vi "Main v1.8.vi"() -> ()   [LabVIEW 2017]
doc: "v0.85:\n- Counts for rejects and total\n\nv0.5:\n\n- Added Reject to Manual Mode\n- Send reject pallet cluster during manual mode\n- Run continuous manual happens only when no error has occured"
uses:
  Controls/Main Tabs v0.1.ctl
  Controls/Auto.ctl
  RT/Controls/Auto Delays.ctl
  RT/Controls/Auto Times.ctl
  support/Controls/General Para.ctl
  Controls/UI Data.ctl
  support/Controls/Auto Stats.ctl
  Controls/Logging FGV.ctl
  support/Message Queue/Enqueue Message (Single).vi
  GV/Maintenance GV.vi
  <vilib>/Utility/error.llb/Error Cluster From Error Code.vi
  <vilib>/ErrorRing/Error Ring.xnode
  support/Message Queue/Message Queue.lvlib
  support/User Event - Stop/User Event - Stop.lvlib
panel:
  out "OEE":dbl format="%#.1f"
  out "QUA":dbl=100.0 min=0.0 max=100.0 step=0.1
  in  "Ideal Time":dbl=2.0 min=0.0 max=100.0 step=0.1
  in  "AVL":dbl=100.0 min=0.0 max=100.0 step=0.1
  out "PRF":dbl=100.0 min=0.0 max=100.0 step=0.1
  out "path":path
  in  "General Para 2":T1={"Max. Cons."=5.0, "Offset 1"=0.0, "Offset 2"=0.0, "Offset 3"=0.0, "Offset 4"=-0.6, "OutputPause"=500.0, "RejectPause"=500.0} caption="General Para" {"Offset 4" format="%.2f"; "Offset 3" format="%.2f"; "Offset 2" format="%.2f"; "Offset 1" format="%.2f"}
  in  "Auto Para 2":T2={"Agitator Delays"=[250, 600], "TF Delays"=[400, 800, 2, 8000], "Insertion Delays"=[100, 400], "Cutting Delays"=[200, 300, 50], "PF Delays"=[300, 8000], "Measur. Delays"=[200.0, 188.9, 1.0], "Reject Delays"=[500], "BF Delays"=[1000, 1000]}
  out "Shutdown?":bool
  in  "Reject Pallets":T3
  out "Date-Time":string caption="Dip-Tube Assembly Automation (HMI) v1.6"
  out "Main Tab":T4
  in  "All IOs":bool
  in  "Autocycle":T5
  in  "Manual":bool
  in  "Parameters":bool
  in  "Maintenance":bool
  in  "General Para":T1={"Max. Cons."=5.0, "Offset 1"=0.0, "Offset 2"=0.0, "Offset 3"=0.0, "Offset 4"=0.0, "OutputPause"=0.0, "RejectPause"=0.0} {"Offset 4" format="%.2f"; "Offset 3" format="%.2f"; "Offset 2" format="%.2f"; "Offset 1" format="%.2f"}
  in  "BF Para":cluster{"Delay 1":u32, "Delay 2":u32}={"Delay 1"=1000, "Delay 2"=1000}
  in  "Reject Para":cluster{"Delay":u32}={"Delay"=400}
  in  "PF Para":cluster{"Delay 1":u32, "Delay 2":u32}={"Delay 1"=1000, "Delay 2"=1000}
  in  "Tube Feeder Para":T6={"Delay"=400, "Delay 2"=250, "Max Attempts"=250, "Timeout"=8000} caption="TF Para"
  in  "Agitator Para":cluster{"Delay 1":u32, "Delay 2":u32}={"Delay 1"=400, "Delay 2"=250}
  in  "Insertion Para":cluster{"Delay 1":u32, "Delay 2":u32}={"Delay 1"=1000, "Delay 2"=1000}
  in  "Save Para":bool
  in  "Home Para":bool
  in  "Cutting Para":T7={"Delay"=400, "Delay 2"=250, "Delay 3"=250}
  in  "Meas. Para":T8={"Delay"=500.0, "Mean Length"=188.9, "Tolerance"=1.0}
  out "Rejects 2":u32 caption="Rejects"
  in  "Reset MCount":bool
  in  "Enable BF?":bool
  in  "Enable Agitate?":bool
  in  "Enable Reject?":bool
  in  "Toggle Motor":bool
  in  "Continuous?":bool
  in  "Enable Measure?":bool
  in  "Enable Index?":bool
  in  "Enable PF?":bool
  in  "Manual Para":T2={"Agitator Delays"=[400, 250], "TF Delays"=[700, 800, 2], "Insertion Delays"=[100, 500], "Cutting Delays"=[300, 300, 100], "PF Delays"=[250, 30000], "Measur. Delays"=[500.0, 188.9, 1.0], "Reject Delays"=[500], "BF Delays"=[1000, 1000]}
  in  "Enable Cutting?":bool
  in  "Enable Insertion?":bool
  in  "Run Manual":bool
  in  "Enable TF?":bool
  in  "Home Manual":bool
  out "Status 2":T10
  out "Measurements":T11 {"Height 1" format="%#.2f"; "Height 2" format="%#.2f"; "Height 3" format="%#.2f"; "Height 4" format="%#.2f"}
  out "Output Count":u32 caption="Output\nCount"
  in  "ResetRejectCount":bool
  in  "ResetGoodCount":bool
  out "RejectPause":u32 caption="Reject Parts"
  out "GoodPause":u32 caption="Good Parts"
  in  "End Cycle":bool
  out "Statuses":string[][](table)
  in  "All IO":bool
  in  "Stats":bool
  in  "Home AC":bool
  out "Status":string
  out "Good":u32 format="%06.0f"
  out "Cycle Time":dbl format="%0.2f"
  out "Rejects":u32 format="%05.0f"
  in  "View Log":bool
  out "Total Count 2":u32 caption="Total Count"
  out "Avg. Time":dbl caption="Avg. Cycle Time (s)" format="%#.3f"
  out "Output Chart":cluster{"Good Parts":u32, "Reject Parts":u32}(graph)
  out "Reject Count":u32
  out "Good Count":u32
  out "Total Time":dbl caption="Effective Cycle Time (s)" format="%#.3f"
  out "Time Chart":T12(graph)
  out "OEE Chart":T13(graph)
  out "Timestamp":string caption="Date & Timestamp"
  out "Latest Measure.":T14 caption="Latest Measurements" {"Length 1 (mm)" format="%#.2f"}
  out "Auto Times":T9
  in  "Back Stats":bool
  out "OEE 2":T13 caption="Latest Measurements" {"AVL" format="%#.1f"; "PRF" format="%#.1f"; "QUA" format="%#.1f"; "OEE" format="%#.1f"}
  out "Measurement Chart":T15(graph)
  in  "Home IOs":bool
  in  "Back IO":bool
  out "IAS 4":dbl format="%#.3f"
  out "IAS 3":dbl format="%#.3f"
  out "IAS 2":dbl format="%#.3f"
  out "IAS 1":dbl format="%#.3f"
  out "DI 1":T16
  out "DI 2":T17
  out "DO 1":T18
  in  "Exit":bool
  in  "Shutdown":bool
  # "HARMONY VISION DIP-TUBE ASSEMBLY AUTOMATION"
  # "Info"
  # "Delays: Time to wait (in milliseconds) after each action pertaining to each spcific station. Generally this timer starts after the required sensor that is expected either goes OFF or goes ON depending on the action. Some stations have multiple delays which are denoted by numbers relative to the sequence of action before the delay.\n\nTimeout: Maximum time allowed (in milliseconds) for a station to complete its actions.\n\nMax Attempts: Maximum number of attempts at retrying gate open/close.\n\nMean Length: Mean length of parts in the current model (in mm)\n\nTolerance: Acceptable deviation from mean length (in mm)\n\nMax Cons.: Maximum number of consecutive tubes missing on a particular pallet (as detected on measurement station) that will trigger an error and cycle stop.\n\nOffset: Offset factor (in mm) added to the measurement result of each probe.\n\nOutputPause & RejectPause: Countdown of number of parts before triggering an Auto-Pause."
  # "Auto-Pause after"
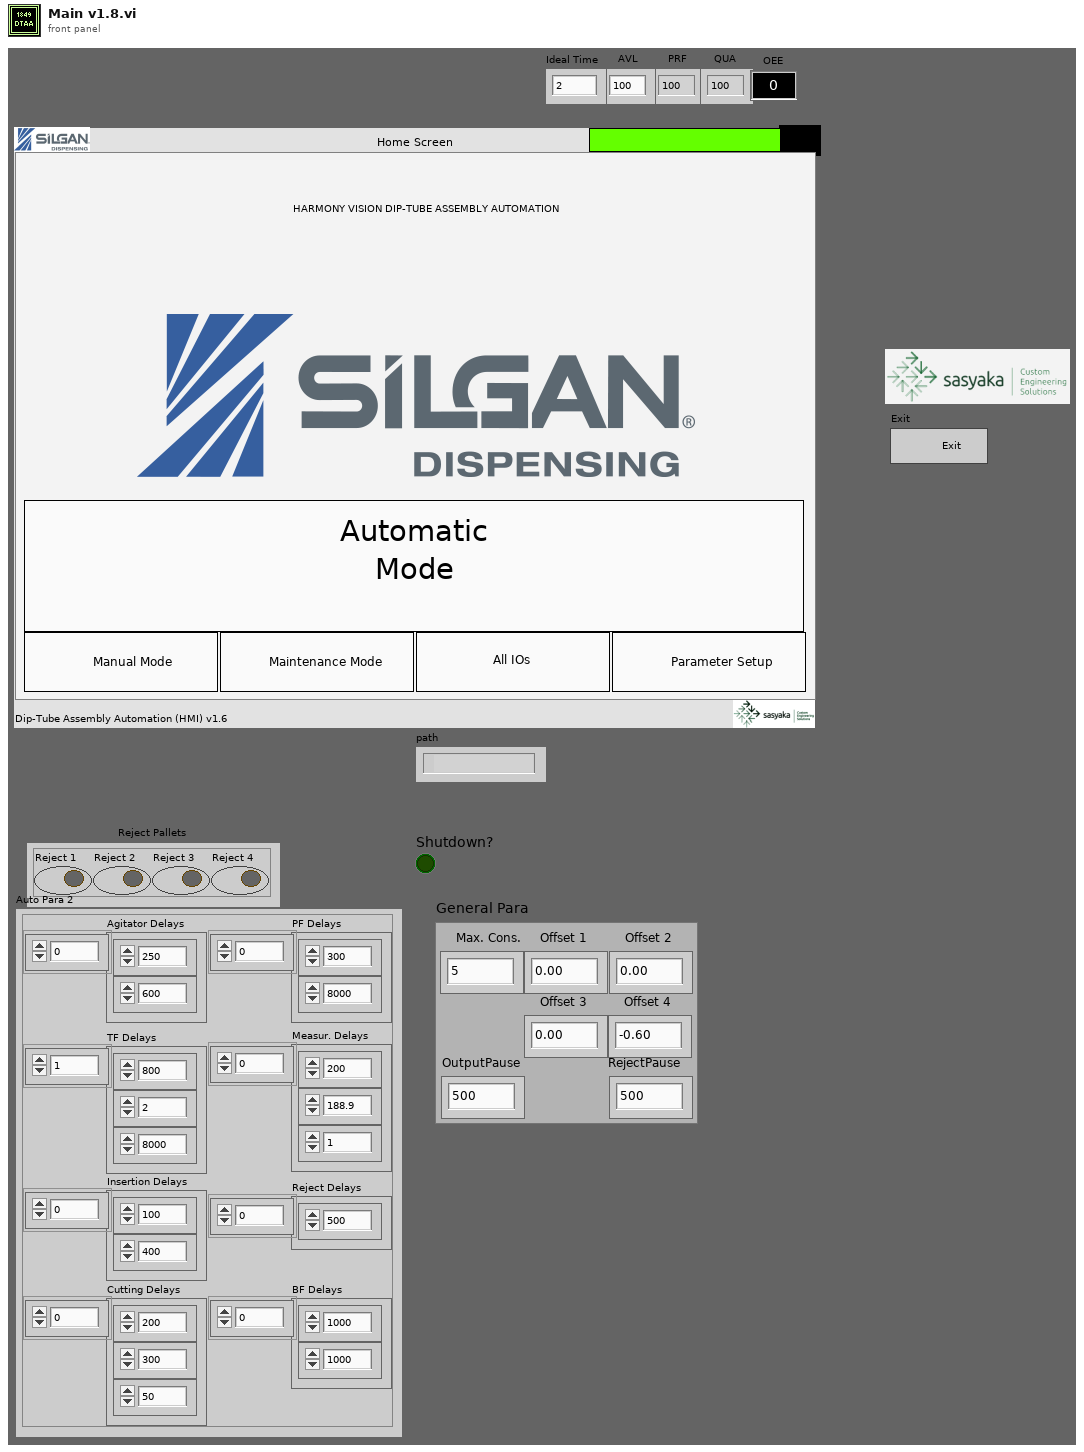
[diagram p1: front panel]
types:
  T1 = typedef "General Para.ctl" = cluster{"Max. Cons.":dbl, "Offset 1":dbl, "Offset 2":dbl, "Offset 3":dbl, "Offset 4":dbl, "OutputPause":dbl, "RejectPause":dbl}
  T2 = typedef "Auto Delays.ctl" = cluster{"Agitator Delays":u32[], "TF Delays":u32[], "Insertion Delays":u32[], "Cutting Delays":u32[], "PF Delays":u32[], "Measur. Delays":dbl[], "Reject Delays":u32[], "BF Delays":u32[]}
  T3 = cluster{"Reject 1":bool, "Reject 2":bool, "Reject 3":bool, "Reject 4":bool}
  T4 = typedef "Main Tabs v0.1.ctl" = enum32{"Home Screen", "Parameter Setup", "Manual Mode", "Autocycle", "Autocycle Statistics", "Autocycle IOs"}
  T5 = typedef "Auto.ctl" = bool
  T6 = cluster{"Delay":u32, "Delay 2":u32, "Max Attempts":u32, "Timeout":u32}
  T7 = cluster{"Delay":u32, "Delay 2":u32, "Delay 3":u32}
  T8 = cluster{"Delay":dbl, "Mean Length":dbl, "Tolerance":dbl}
  T9 = typedef "Auto Times.ctl" = cluster{"Index Time":u32, "TF Time":u32, "Insertion Time":u32, "Cutting Time":u32, "PF Time":u32, "Meas. Time":u32, "Reject Time":u32}
  T10 = cluster{"Auto Times":T9, "error out":errorcluster}
  T11 = cluster{"Height 1":dbl, "Height 2":dbl, "Height 3":dbl, "Height 4":dbl}
  T12 = cluster{"Index":dbl, "TF":dbl, "Insert":dbl, "Cutting":dbl, "PF":dbl, "Measure.":dbl, "Reject":dbl, "Avg. Cycle Time":dbl}
  T13 = cluster{"AVL":dbl, "PRF":dbl, "QUA":dbl, "OEE":dbl}
  T14 = cluster{"Length 1 (mm)":dbl, "Pallet 2 (mm)":dbl, "Pallet 3 (mm)":dbl, "Pallet 4 (mm)":dbl}
  T15 = cluster{"1":dbl, "2":dbl, "3":dbl, "4":dbl, "4":dbl, "4":dbl}
  T16 = cluster{"Machine_ON":bool, "E_stop ":bool, "SW_Pressure":bool, "SW_Start ":bool, "SW_Reset":bool, "SW_Stop":bool, "SW_Door":bool, "RS_Index_Rotary_CW":bool, "RS_Index_Rotary_CCW":bool, "RS_Index_Stopper _Rear":bool, "RS_Index_Output_Separator_Rear":bool, "PES_Index_Pallet_Sensor":bool, "PES_Index_Output_Part Sensor":bool, "ICS_BF_Low_Level_1":bool, "ICS_BF_Low_Level_2":bool, "ICS_BF_Pump_CNVR_Full_1":bool, "ICS_BF_Pump_CNVR_Full_2":bool, "ICS_BF_Pump_CNVR_Full_3":bool, "ICS_BF_Pump_CNVR_Full_4":bool, "PES_PC_Pump Presence_1":bool, "PES_PC_Pump Presence_2":bool, "PES_PC_Pump Presence_3":bool, "PES_PC_Pump Presence_4":bool, "RS_PC_Gating_Front":bool, "PES_Pump_Interference":bool, "PES_TF_Low_Level":bool, "PES_Tube Presence_1":bool, "PES_Tube Presence_2":bool, "PES_Tube Presence_3":bool, "PES_Tube Presence_4":bool, "DI1.30":bool, "DI1.31":bool}
  T17 = cluster{"RS_Agitatator_1_Rear ":bool, "RS_Agitatator_2_Rear ":bool, "RS_TF_Gating CYL_Rear":bool, "RS_Insertion_1_Rear":bool, "RS_Insertion_1_Front":bool, "RS_Insertion _2_Rear":bool, "RS_Insertion _2_Front":bool, "RS_Insertion _3_Rear":bool, "RS_Insertion _3_Front":bool, "RS_Insertion _4_Rear":bool, "RS_Insertion _4_Front":bool, "RS_Insertion_Clamp_Rear":bool, "RS_Cutting_Rear":bool, "RS_Cutting_Clamp _Rear":bool, "RS_Measurement_1_Rear":bool, "RS_Measurement_2_Rear":bool, "RS_Measurement_3_Rear":bool, "RS_Measurement_4_Rear":bool, "DI2.18":bool, "RS_Rejection_1_Rear":bool, "RS_Rejection_2_Rear":bool, "RS_Rejection_3_Rear":bool, "RS_Rejection_4_Rear":bool, "DI2.23":bool, "DI2.24":bool, "DI2.25":bool, "DI2.26":bool, "DI2.27":bool, "DI2.28":bool, "DI2.29":bool, "DI2.30":bool, "DI2.31":bool}
  T18 = cluster{"TL_Red":bool, "TL_Orange":bool, "TL_Green":bool, "TL_Buzzer":bool, "SOL_Index_Rotary_CW":bool, "SOL_Index_Rotary_CCW":bool, "SOL_Index_Stopper_Rear":bool, "SOL_OutputSeparator_Rear":bool, "Bowl  Feeder_ ON 1":bool, "Pump_CNVR_Motor _ON":bool, "SOL_PC_Gating_CYL_Rear":bool, "SOL_Tube_Feed_Agitatator":bool, "SOL_Tube_Feed_Gating_CYL":bool, "SOL_Insertion _CYL":bool, "SOL_Insertion_Clamp_CYL":bool, "SOL_Cutting_CYL":bool, "SOL_Cutting_Clamp_CYL":bool, "SOL_Insertion_Air_Nozzle":bool, "SOL_Measurement_CYL":bool, "DO1.19":bool, "SOL_Rejection CYL_1":bool, "SOL_Rejection CYL_2":bool, "SOL_Rejection CYL_3":bool, "SOL_Rejection CYL_4":bool, "Bowl  Feeder_ ON 2":bool, "SOL_BF_BlowerON":bool, "SOL_BF1_Track1":bool, "SOL_BF1_Track2":bool, "SOL_BF2_Track1":bool, "SOL_BF2_Track2":bool, "DO1.30":bool, "DO1.31":bool}
  T19 = typedef "UI Data.ctl" = cluster{"Main Tab":refnum<vi>}
  T20 = typedef "Message Queue.lvlib/All Message Queues.ctl" = cluster{"UI":refnum<queue>}
  T21 = enum8{"Enabled", "Disabled", "Disabled and Grayed Out"}
  T22 = cluster{"Array":string[][], "Machine Status":string}
  T23 = typedef "Logging FGV.ctl" = enum16{"Start Shift", "Log Index", "Read Shift", "Close Shift"}
  T24 = typedef "Auto Stats.ctl" = cluster{"Time-Stamp":timestamp, "Auto Times":T9, "Measurements":cluster{"1":dbl, "2":dbl, "3":dbl, "4":dbl}, "Outputs":cluster{"Good Parts":u32, "Reject Parts":u32}, "Cycle Time":dbl, "Remarks":string}
  T25 = cluster{"Auto Times":T9, "Results":cluster{"Measurements":cluster{"1":dbl, "2":dbl, "3":dbl, "4":dbl}, "Reject Pallets":cluster{"Reject 1":bool, "Reject 2":bool, "Reject 3":bool, "Reject 4":bool}}, "OutputCount":u32, "error out":errorcluster}
  T26 = enum8{"Information", "Error", "Successful", "Tips"}
  T27 = cluster{"Agitator Delays[0]":u32, "Agitator Delays[1]":u32}
  T28 = cluster{"TF Delays[0]":u32, "TF Delays[1]":u32, "TF Delays[2]":u32, "TF Delays[3]":u32}
  T29 = cluster{"Insertion Delays[0]":u32, "Insertion Delays[1]":u32}
  T30 = cluster{"Cutting Delays[0]":u32, "Cutting Delays[1]":u32, "Cutting Delays[2]":u32}
  T31 = cluster{"Measur. Delays[0]":dbl, "Measur. Delays[1]":dbl, "Measur. Delays[2]":dbl}
  T32 = typedef "All Inputs.ctl" = cluster{"DI 1":cluster{"Machine_ON":bool, "E_stop ":bool, "SW_Pressure":bool, "SW_Start ":bool, "SW_Reset":bool, "SW_Stop":bool, "SW_Door":bool, "RS_Index_Rotary_CW":bool, "RS_Index_Rotary_CCW":bool, "RS_Index_Stopper _Rear":bool, "RS_Cutting_DNClamp _Rear":bool, "PES_Index_Pallet_Sensor":bool, "PES_Index_Output_Part Sensor":bool, "ICS_BF_Low_Level_1":bool, "ICS_BF_Low_Level_2":bool, "ICS_BF_Pump_CNVR_Full_1":bool, "ICS_BF_Pump_CNVR_Full_2":bool, "ICS_BF_Pump_CNVR_Full_3":bool, "ICS_BF_Pump_CNVR_Full_4":bool, "PES_PC_Pump Presence_1":bool, "PES_PC_Pump Presence_2":bool, "PES_PC_Pump Presence_3":bool, "PES_PC_Pump Presence_4":bool, "RS_PC_Gating_Front":bool, "PES_Pump_Interference":bool, "PES_TF_Low_Level":bool, "PES_Tube Presence_1":bool, "PES_Tube Presence_2":bool, "PES_Tube Presence_3":bool, "PES_Tube Presence_4":bool, "DI1.30":bool, "DI1.31":bool}, "DI 2":cluster{"RS_Agitatator_1_Rear ":bool, "RS_Agitatator_2_Rear ":bool, "RS_TF_Gating CYL_Rear":bool, "RS_Insertion_1_Rear":bool, "RS_Insertion_1_Front":bool, "RS_Insertion _2_Rear":bool, "RS_Insertion _2_Front":bool, "RS_Insertion _3_Rear":bool, "RS_Insertion _3_Front":bool, "RS_Insertion _4_Rear":bool, "RS_Insertion _4_Front":bool, "RS_Insertion_Clamp_Rear":bool, "RS_Cutting_Rear":bool, "RS_Cutting_UPClamp _Rear":bool, "RS_Measurement_1_Rear":bool, "RS_Measurement_2_Rear":bool, "RS_Measurement_3_Rear":bool, "RS_Measurement_4_Rear":bool, "RS_Measure_Clamp_Rear":bool, "RS_Rejection_1_Rear":bool, "RS_Rejection_2_Rear":bool, "RS_Rejection_3_Rear":bool, "RS_Rejection_4_Rear":bool, "DI2.23":bool, "DI2.24":bool, "DI2.25":bool, "DI2.26":bool, "DI2.27":bool, "DI2.28":bool, "DI2.29":bool, "DI2.30":bool, "DI2.31":bool}, "IAS 1":dbl, "IAS 2":dbl, "IAS 3":dbl, "IAS 4":dbl, "DO 1":cluster{"TL_Red":bool, "TL_Orange":bool, "TL_Green":bool, "TL_Buzzer":bool, "SOL_Index_Rotary_CW":bool, "SOL_Index_CNVR_Rotary_CCW":bool, "SOL_Index_CNVR_Stopper_Rear":bool, "SOL_Index_CNVR_Output _Separator _Rear":bool, "Bowl  Feeder_ ON 1":bool, "Pump_CNVR_Motor _ON":bool, "SOL_PC_Gating_CYL_Rear":bool, "SOL_Tube_Feed_Agitatator":bool, "SOL_Tube_Feed_Gating_CYL":bool, "SOL_Insertion _CYL":bool, "SOL_Insertion_Clamp_CYL":bool, "SOL_Cutting_CYL":bool, "SOL_Cutting_Clamp_CYL":bool, "SOL_Insertion_Air_Nozzle":bool, "SOL_Measurement_CYL":bool, "DO1.19":bool, "SOL_Rejection CYL_1":bool, "SOL_Rejection CYL_2":bool, "SOL_Rejection CYL_3":bool, "SOL_Rejection CYL_4":bool, "Bowl  Feeder_ ON 2":bool, "SOL_BF_BlowerON":bool, "SOL_BF1_Track1":bool, "SOL_BF1_Track2":bool, "SOL_BF2_Track1":bool, "SOL_BF2_Track2":bool, "DO1.30":bool, "DO1.31":bool}}
  T33 = cluster{"Machine_ON":bool, "E_stop ":bool, "SW_Pressure":bool, "SW_Start ":bool, "SW_Reset":bool, "SW_Stop":bool, "SW_Door":bool, "RS_Index_Rotary_CW":bool, "RS_Index_Rotary_CCW":bool, "RS_Index_Stopper _Rear":bool, "RS_Cutting_DNClamp _Rear":bool, "PES_Index_Pallet_Sensor":bool, "PES_Index_Output_Part Sensor":bool, "ICS_BF_Low_Level_1":bool, "ICS_BF_Low_Level_2":bool, "ICS_BF_Pump_CNVR_Full_1":bool, "ICS_BF_Pump_CNVR_Full_2":bool, "ICS_BF_Pump_CNVR_Full_3":bool, "ICS_BF_Pump_CNVR_Full_4":bool, "PES_PC_Pump Presence_1":bool, "PES_PC_Pump Presence_2":bool, "PES_PC_Pump Presence_3":bool, "PES_PC_Pump Presence_4":bool, "RS_PC_Gating_Front":bool, "PES_Pump_Interference":bool, "PES_TF_Low_Level":bool, "PES_Tube Presence_1":bool, "PES_Tube Presence_2":bool, "PES_Tube Presence_3":bool, "PES_Tube Presence_4":bool, "DI1.30":bool, "DI1.31":bool}
  T34 = cluster{"RS_Agitatator_1_Rear ":bool, "RS_Agitatator_2_Rear ":bool, "RS_TF_Gating CYL_Rear":bool, "RS_Insertion_1_Rear":bool, "RS_Insertion_1_Front":bool, "RS_Insertion _2_Rear":bool, "RS_Insertion _2_Front":bool, "RS_Insertion _3_Rear":bool, "RS_Insertion _3_Front":bool, "RS_Insertion _4_Rear":bool, "RS_Insertion _4_Front":bool, "RS_Insertion_Clamp_Rear":bool, "RS_Cutting_Rear":bool, "RS_Cutting_UPClamp _Rear":bool, "RS_Measurement_1_Rear":bool, "RS_Measurement_2_Rear":bool, "RS_Measurement_3_Rear":bool, "RS_Measurement_4_Rear":bool, "RS_Measure_Clamp_Rear":bool, "RS_Rejection_1_Rear":bool, "RS_Rejection_2_Rear":bool, "RS_Rejection_3_Rear":bool, "RS_Rejection_4_Rear":bool, "DI2.23":bool, "DI2.24":bool, "DI2.25":bool, "DI2.26":bool, "DI2.27":bool, "DI2.28":bool, "DI2.29":bool, "DI2.30":bool, "DI2.31":bool}
  T35 = cluster{"TL_Red":bool, "TL_Orange":bool, "TL_Green":bool, "TL_Buzzer":bool, "SOL_Index_Rotary_CW":bool, "SOL_Index_CNVR_Rotary_CCW":bool, "SOL_Index_CNVR_Stopper_Rear":bool, "SOL_Index_CNVR_Output _Separator _Rear":bool, "Bowl  Feeder_ ON 1":bool, "Pump_CNVR_Motor _ON":bool, "SOL_PC_Gating_CYL_Rear":bool, "SOL_Tube_Feed_Agitatator":bool, "SOL_Tube_Feed_Gating_CYL":bool, "SOL_Insertion _CYL":bool, "SOL_Insertion_Clamp_CYL":bool, "SOL_Cutting_CYL":bool, "SOL_Cutting_Clamp_CYL":bool, "SOL_Insertion_Air_Nozzle":bool, "SOL_Measurement_CYL":bool, "DO1.19":bool, "SOL_Rejection CYL_1":bool, "SOL_Rejection CYL_2":bool, "SOL_Rejection CYL_3":bool, "SOL_Rejection CYL_4":bool, "Bowl  Feeder_ ON 2":bool, "SOL_BF_BlowerON":bool, "SOL_BF1_Track1":bool, "SOL_BF1_Track2":bool, "SOL_BF2_Track1":bool, "SOL_BF2_Track2":bool, "DO1.30":bool, "DO1.31":bool}
  T36 = cluster{"Index":dbl, "TF":dbl, "Insert":dbl, "Cutting":dbl, "PF":dbl, "Measure.":dbl, "Reject":dbl}
  T37 = cluster{"1":dbl, "2":dbl, "3":dbl, "4":dbl, dbl, dbl}
  T38 = cluster{"Manual Para":T2, "Reject Pallets":cluster{"Reject 1":bool, "Reject 2":bool, "Reject 3":bool, "Reject 4":bool}}
  T39 = cluster{"Measurements":cluster{"1":dbl, "2":dbl, "3":dbl, "4":dbl}, "Reject Pallets":cluster{"Reject 1":bool, "Reject 2":bool, "Reject 3":bool, "Reject 4":bool}}
  T40 = cluster{"Reject Pallets":cluster{"Reject 1":bool, "Reject 2":bool, "Reject 3":bool, "Reject 4":bool}, "Measurements":cluster{"1":dbl, "2":dbl, "3":dbl, "4":dbl}}
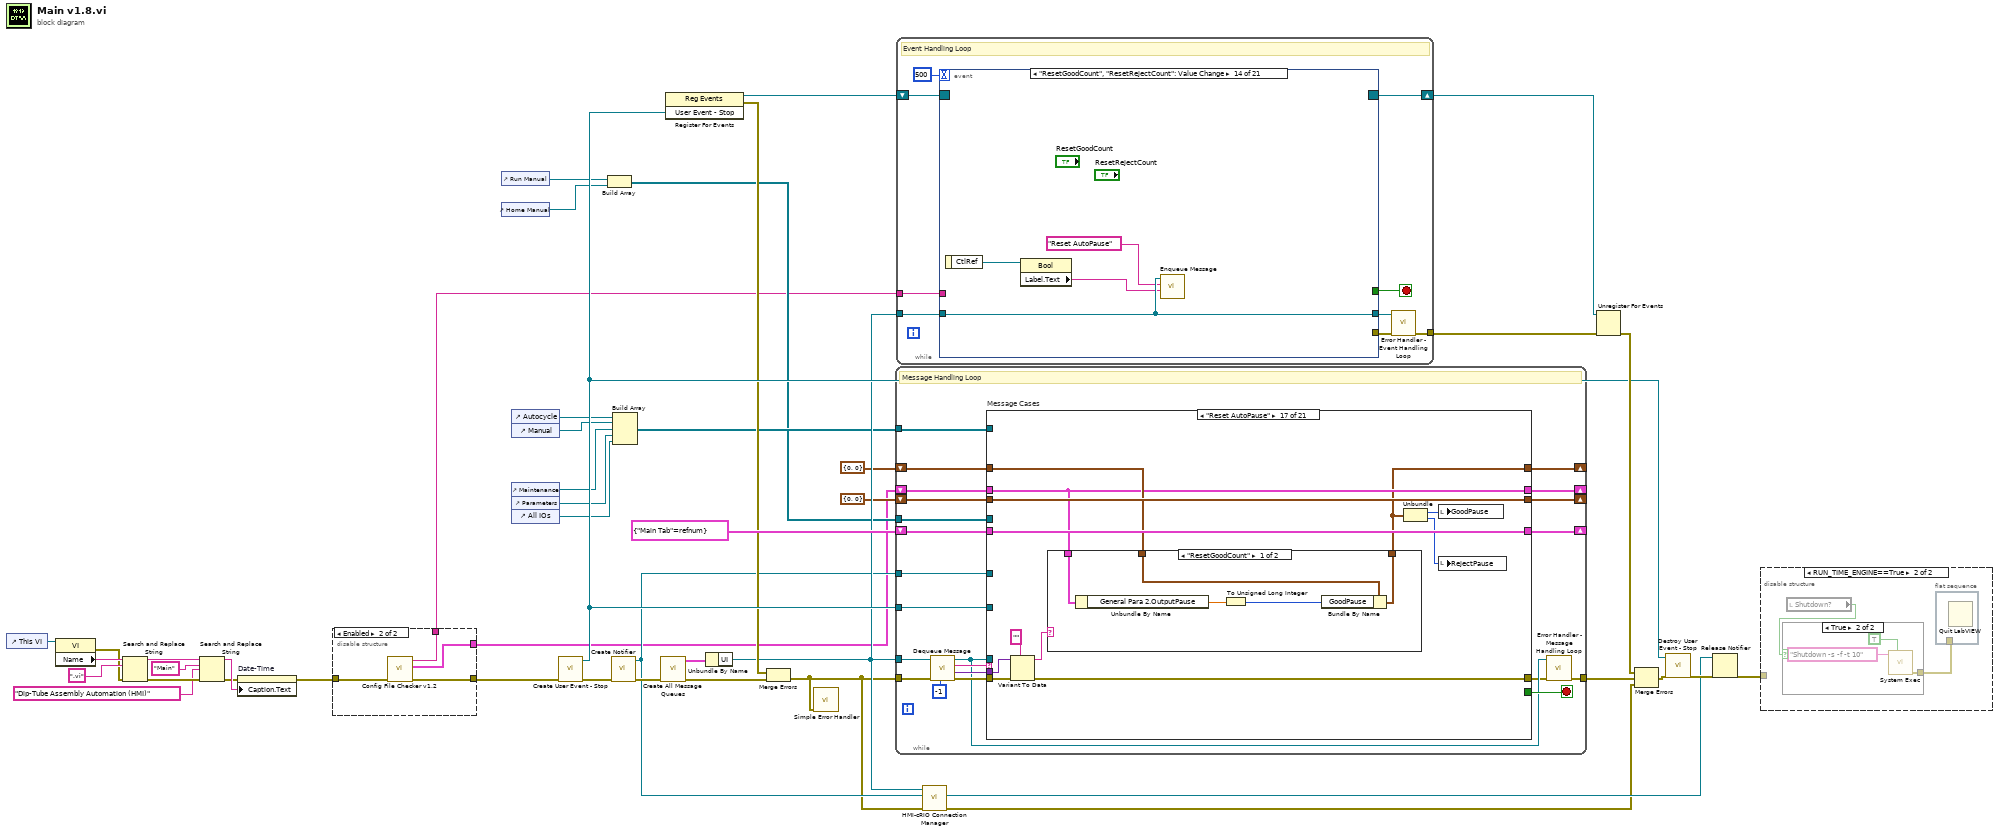
[diagram p0: block diagram]
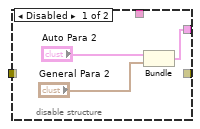
[diagram p2: hidden frame]
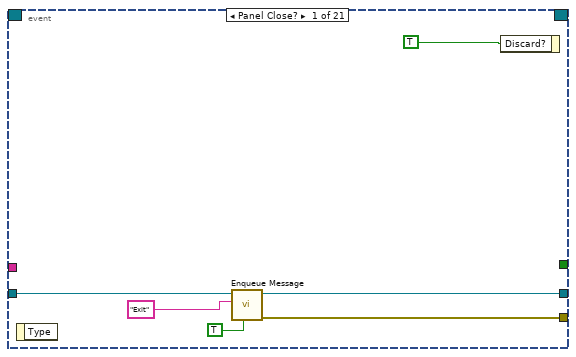
[diagram p3: hidden frame]
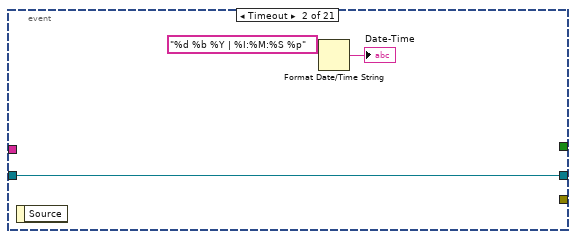
[diagram p4: hidden frame]
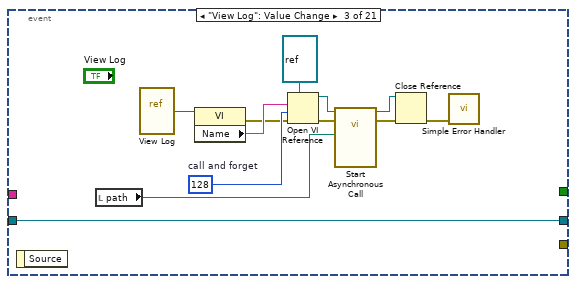
[diagram p5: hidden frame]
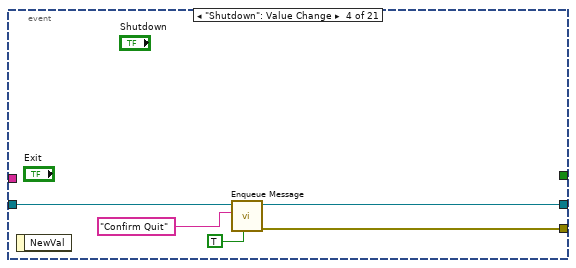
[diagram p6: hidden frame]
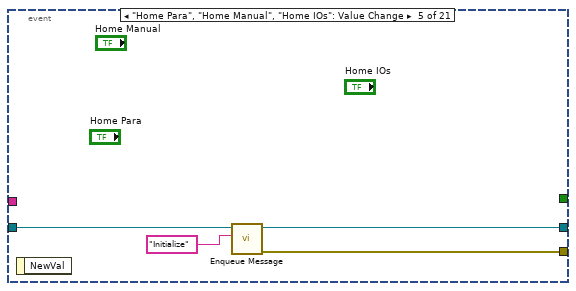
[diagram p7: hidden frame]
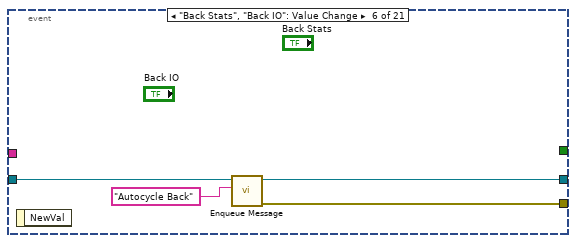
[diagram p8: hidden frame]
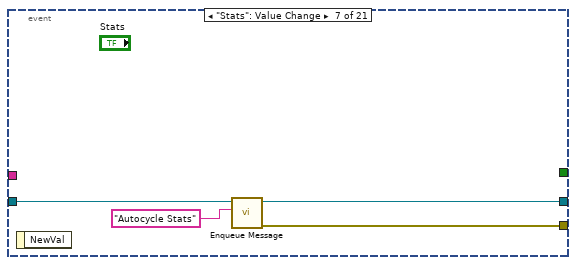
[diagram p9: hidden frame]
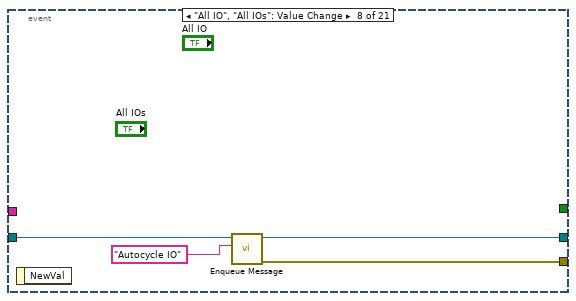
[diagram p10: hidden frame]
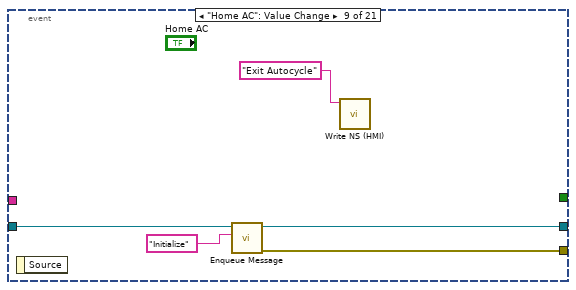
[diagram p11: hidden frame]
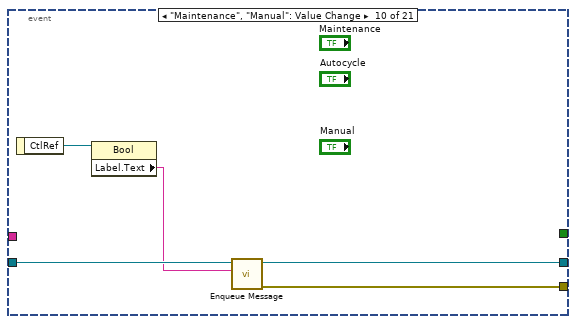
[diagram p12: hidden frame]
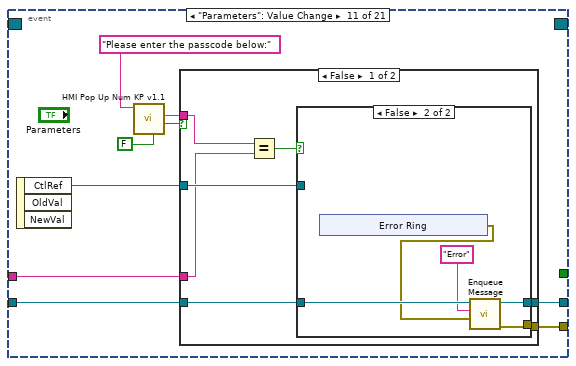
[diagram p13: hidden frame]
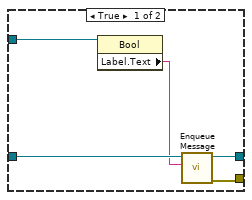
[diagram p14: hidden frame]
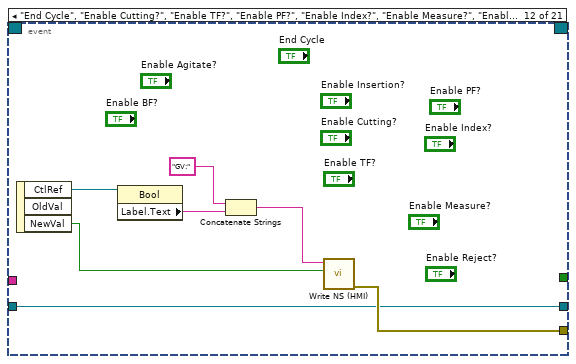
[diagram p16: hidden frame]
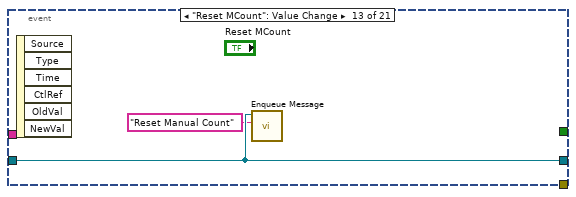
[diagram p17: hidden frame]
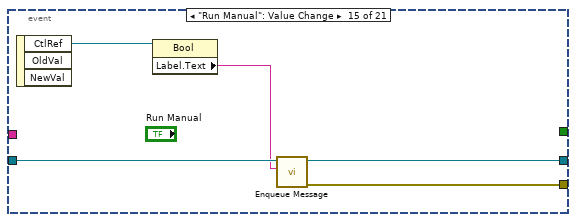
[diagram p18: hidden frame]
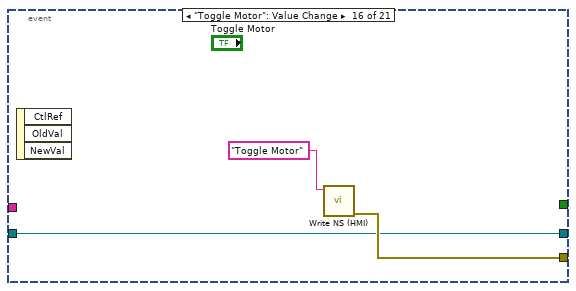
[diagram p19: hidden frame]
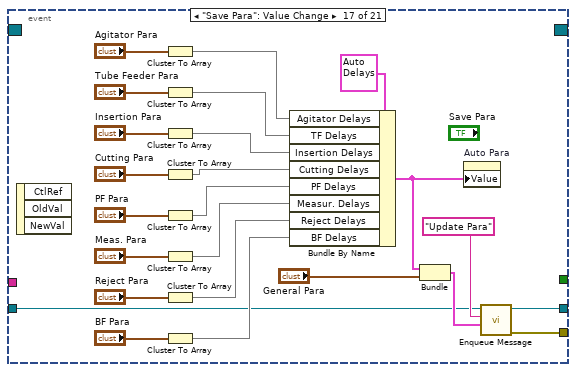
[diagram p20: hidden frame]
diagram:
  n1 = control-ref of="This VI"() -> (w16:refnum<vi>)
  n2 = property class="VI"(reference=w16) -> (error out=w15:errorcluster, "Name"=w22:string)  [unwired: 1 in, 1 out]
  n3 = Search and Replace String(input string=w22, search string=".vi", error in=w15) -> (result string=w20:string, error out=w19:errorcluster)  [unwired: 5 in, 2 out]
  n4 = Search and Replace String(input string=w20, search string="Main", replace string="Dip-Tube Assembly Automation (HMI)" ("replace string (\"\")"), error in=w19) -> (result string=w14:string, error out=w13:errorcluster)  [unwired: 4 in, 2 out]
  n5 = property on="Date-Time" class="Str"(error in=w13, "Caption.Text"=w14) -> (error out=w6:errorcluster)  [unwired: 1 in, 1 out]
  n6 = disable-structure shown="Enabled" {
    disable-tunnel: [w46 w52] -> w4
    disable-tunnel: w6 -> [_ w51]
    disable-tunnel: [_ w50] -> w5
    disable-tunnel: [_ w49] -> w3
    frame Disabled {
      n7 = Bundle("Auto Para 2"="Auto Para 2", "General Para 2"="General Para 2") -> (w46:cluster{"Auto Para 2":T2, "General Para 2":T1})  [unwired: 1 in]
    }
    frame Enabled {
      n8 = call "Config File Checker v1.2.vi"("Error In"=w51) -> ("error out"=w50:errorcluster, "All Para"=w52:cluster{"Auto Para":T2, "General Para 2":T1}, "password"=w49:string)  [unwired: 7 in, 1 out]
    }
  }
  n9 = control-ref of="Run Manual"() -> (w12:refnum<vi>)
  n10 = control-ref of="Home Manual"() -> (w11:refnum<vi>)
  n11 = control-ref of="Autocycle"() -> (w27:refnum<vi>)
  n12 = control-ref of="Manual"() -> (w26:refnum<vi>)
  n13 = control-ref of="Maintenance"() -> (w25:refnum<vi>)
  n14 = control-ref of="Parameters"() -> (w24:refnum<vi>)
  n15 = control-ref of="All IOs"() -> (w7:refnum<vi>)
  n16 = call "Create User Event - Stop.vi"("error in (no error)"=w5) -> ("error out"=w33:errorcluster, "User Event - Stop"=w36:refnum<user-event>)  [unwired: 9 in]
  n17 = Build Array(w12, w11) -> (w10:refnum<vi>[])
  n18 = call "Create Notifier.vi"("error in (no error)"=w33) -> ("error out"=w32:errorcluster, "notifier out"=w8:refnum<notifier>)  [unwired: 9 in]
  n19 = Build Array(w27, w26, w25, w24, w7) -> (w23:refnum<vi>[])
  n20 = call "Create All Message Queues.vi"("error in (no error)"=w32) -> ("error out"=w45:errorcluster, "Message Queues out"=w44:T20)  [unwired: 9 in]
  n21 = register-events(w36) -> (reference out=w37:refnum<event-registration>, error out=w35:errorcluster)  [unwired: 2 in]
  n22 = Unbundle By Name(w44) -> ("UI"=w34:refnum<queue>)
  n23 = Merge Errors(w35, w45) -> (w2:errorcluster)
  n24 = call <vilib>:"Simple Error Handler.vi"("error in (no error)"=w2) -> ()  [unwired: 4 in, 5 out]
  n25 = while {
    tunnel: w34 -> [w67]
    shift-right: [w74] -> _
    shift-left: T19 {"Main Tab"=refnum} ("Data Cluster") -> [w57]
    tunnel: w36 -> [w72]
    tunnel: w2 -> [w71]
    tunnel: [w65] -> w43
    tunnel: w8 -> [w62]
    tunnel: w23 -> [w61]
    tunnel: w10 -> [w60]
    shift-right: [w58] -> _
    shift-left: cluster{"OutputCount":u32, "RejectCount":u32} {"OutputCount"=0, "RejectCount"=0} -> [w59]
    shift-right: [w55] -> _
    shift-left: w4 -> [w56]
    shift-right: [w53] -> _
    shift-left: cluster{"GoodPause":u32, "RejectPause":u32} {"GoodPause"=0, "RejectPause"=0} ("cluster") -> [w54]
    stop <- w73 stop-if-true
    # "Message Handling Loop"
    n26 = call "Dequeue Message.vi"("timeout"=-1, "error in (no error)"=w71, "Message Queue"=w67) -> ("error out"=w70:errorcluster, "Message Data"=w68:variant, "Message"=w69:string, "dup Message Queue"=w66:refnum<queue>)  [unwired: 5 in]
    n27 = case "Message Cases" shown="\"Reset AutoPause\"" w69 {
      selector: w69 -> [_ _ _ _ _ _ _ _ _ _ _ _ _ _ _ _ _ _ _ _ w469]
      tunnel: w66 -> [_ _ _ _ _ _ _ _ _ w225 w235 _ w280 _ w361 _ _ _ w438 w465 _]
      tunnel: w70 -> [w84 w89 w105 w135 w152 w170 w181 w211 w218 w227 w243 w273 w323 w335 w369 w381 w391 w428 w442 w458 _]
      tunnel: [w84 w88 w94 w135 w147 w170 w180 w211 w218 w226 w242 w274 w324 w337 w360 w381 w390 w423 w440 w461 w470] -> w64
      tunnel: w57 -> [w83 w90 w107 w139 w154 w169 w177 w215 w222 w232 w240 w275 w325 w338 w370 w380 w393 w427 w441 w464 w471]
      tunnel: [w82 w90 w107 w139 w154 w169 w177 w215 w222 w232 w240 w275 w325 w338 w370 w380 w393 w427 w441 w464 w471] -> w74
      tunnel: [_ _ _ _ _ _ _ _ _ _ _ _ _ _ _ _ _ _ _ TRUE _] -> w73
      tunnel: w68 -> [_ _ w104 _ w151 _ _ _ _ _ _ w272 w322 _ w368 _ w389 w426 _ w455 _]
      tunnel: w72 -> [_ _ _ _ _ _ _ _ _ _ _ _ _ _ _ _ _ _ _ w460 _]
      tunnel: w62 -> [_ _ _ _ _ _ _ _ _ _ _ _ _ _ _ _ _ _ _ w454 _]
      tunnel: w61 -> [_ _ w100 _ _ _ _ _ _ _ _ _ _ _ _ _ _ _ _ _ _]
      tunnel: w60 -> [_ _ _ _ _ _ _ _ _ _ _ _ _ w332 w366 _ _ _ _ _ _]
      tunnel: w59 -> [w79 w87 w96 w136 w153 w158 w182 w212 w219 w229 w244 w270 w320 w328 w359 _ w392 w422 w437 w451 w468]
      tunnel: [w79 w87 w96 w136 w153 w158 w182 w212 w219 w229 w244 w270 w320 w328 w354 cluster{"OutputCount":u32, "RejectCount":u32} {"OutputCount"=0, "RejectCount"=0} w392 w422 w437 w451 w468] -> w58
      tunnel: w56 -> [w76 w86 w93 w116 _ w157 w176 w210 w217 w224 w234 w259 w289 w327 w342 w377 w385 w405 w430 w450 w467]
      tunnel: [w76 w86 w93 w116 w146 w157 w176 w210 w217 w224 w234 w259 w289 w327 w342 w377 w385 w405 w430 w450 w467] -> w55
      tunnel: w54 -> [w75 w85 w91 w115 w140 w155 w173 w209 w216 w223 w233 w258 w281 w326 w341 w376 w386 w404 w429 w449 w466]
      tunnel: [w75 w85 w91 w115 w140 w155 w174 w209 w216 w223 w233 w258 w278 w326 w341 w376 w384 w404 w429 w449 w466] -> w53
      frame "Initialize" {
        # "Initialize - All initialization work should take place in this message, since other loops can potentially enqueue messages that execute immediately after this one."
        n28 = control-ref of="Main Tab"() -> (w81:refnum<vi>)
        n29 = Bundle By Name(cluster=w83, "Main Tab"=w81) -> (w82:T19)
        n30 = property on="Home IOs" class="Bool"("Visible"=TRUE) -> ()  [unwired: 2 in, 2 out]
        n31 = property on="Back IO" class="Bool"("Visible"=FALSE) -> ()  [unwired: 2 in, 2 out]
        "Main Tab" <- Main_Tabs_v0.1."Home Screen" ("Main Tab")
      }
      frame "Maintenance" {
        # "Maintenance"
        n32 = call "Maintenance v0.3.vi"("Error In"=w89) -> ("Error out"=w88:errorcluster)  [unwired: 10 in]
      }
      frame "Connection" {
        n33 = Variant To Data(error in=w105, type=FALSE, Variant=w104) -> (data=w92:bool, error out=w95:errorcluster)
        n34 = Select(t=u32 6618880 ("Text.Text Colors:BG Color"), s=w92, f=u32 16762112 ("Text.Text Colors:BG Color")) -> (s? t:f=w101:u32)
        n35 = property on="Date-Time" class="Str"("Text.BGColor"=w101) -> ()  [unwired: 2 in, 2 out]
        n36 = Select(t=T21."Enabled" ("Disabled"), s=w92, f=T21."Disabled and Grayed Out") -> (s? t:f=w98:T21)
        n37 = for {
          tunnel: w100 -> [w114] mode=indexing
          tunnel: w98 -> [w113]
          n38 = property class="Bool"(reference=w114, "DisabledEnum"=w113) -> ()  [unwired: 1 in, 2 out]
        }
        n39 = case shown="True" w92 {
          tunnel: w95 -> [w108 w111]
          tunnel: [w108 w110] -> w94
          tunnel: w93 -> [_ w109]
          frame False {
          }
          frame True {
            n40 = call "Write NS (HMI).vi"("error in (no error)"=w111, "Message Data"=w109, "Message"="Save Para") -> ("error out"=w110:errorcluster)  [unwired: 8 in]
          }
        }
      }
      frame "Parameters" {
        # "Parameters"
        n41 = Unbundle(w116) -> ("Auto Para"=w118:T2, "General Para 2"=w117:T1)
        n42 = Unbundle By Name(w139) -> ("Main Tab"=w138:refnum<vi>)
        n43 = property on="General Para" class="Clust (strict)"("Value"=w117) -> ()  [unwired: 2 in, 2 out]
        n44 = Unbundle(w118) -> ("Agitator Delays"=w134:u32[], "TF Delays"=w133:u32[], "Insertion Delays"=w132:u32[], "Cutting Delays"=w131:u32[], "PF Delays"=w130:u32[], "Measur. Delays"=w129:dbl[], "Reject Delays"=w128:u32[], "BF Delays"=w127:u32[])
        n45 = property class="TabCtl"(reference=w138, "Value"=Main_Tabs_v0.1."Parameter Setup" ("Main Tab")) -> ()  [unwired: 1 in, 2 out]
        n46 = Array To Cluster(array=w134) -> (cluster=w126:T27)
        n47 = Array To Cluster(array=w133) -> (cluster=w125:T28)
        n48 = Array To Cluster(array=w132) -> (cluster=w124:T29)
        n49 = Array To Cluster(array=w131) -> (cluster=w123:T30)
        n50 = Array To Cluster(array=w130) -> (cluster=w122:cluster{"PF Delays[0]":u32, "PF Delays[1]":u32})
        n51 = Array To Cluster(array=w129) -> (cluster=w121:T31)
        n52 = Array To Cluster(array=w128) -> (cluster=w120:cluster{"Reject Delays[0]":u32})
        n53 = Array To Cluster(array=w127) -> (cluster=w119:cluster{"BF Delays[0]":u32, "BF Delays[1]":u32})
        n54 = property on="Agitator Para" class="Clust (strict)"("Value"=w126) -> ()  [unwired: 2 in, 2 out]
        n55 = property on="Tube Feeder Para" class="Clust (strict)"("Value"=w125) -> ()  [unwired: 2 in, 2 out]
        n56 = property on="Insertion Para" class="Clust (strict)"("Value"=w124) -> ()  [unwired: 2 in, 2 out]
        n57 = property on="Cutting Para" class="Clust (strict)"("Value"=w123) -> ()  [unwired: 2 in, 2 out]
        n58 = property on="PF Para" class="Clust (strict)"("Value"=w122) -> ()  [unwired: 2 in, 2 out]
        n59 = property on="Meas. Para" class="Clust (strict)"("Value"=w121) -> ()  [unwired: 2 in, 2 out]
        n60 = property on="Reject Para" class="Clust (strict)"("Value"=w120) -> ()  [unwired: 2 in, 2 out]
        n61 = property on="BF Para" class="Clust (strict)"("Value"=w119) -> ()  [unwired: 2 in, 2 out]
      }
      frame "Update Para" {
        # "Parameters"
        n62 = Variant To Data(error in=w152, type=cluster{"Auto Para":T2, "General Para":T1} {"Auto Para"={"Agitator Delays"=[], "TF Delays"=[], "Insertion Delays"=[], "Cutting Delays"=[], "PF Delays"=[], "Measur. Delays"=[], "Reject Delays"=[], "BF Delays"=[]}, "General Para"={"Max. Cons."=0.0, "Offset 1"=0.0, "Offset 2"=0.0, "Offset 3"=0.0, "Offset 4"=0.0, "OutputPause"=0.0, "RejectPause"=0.0}} ("cluster"), Variant=w151) -> (data=w146:cluster{"Auto Para":T2, "General Para":T1}, error out=w148:errorcluster)
        n63 = call <vilib>:"Application Directory.vi"() -> ("Application Directory"=w145:path)
        n64 = Build Path(base path=w145, name or relative path="data") -> (appended path=w143:path)
        n65 = Build Path(base path=w143, name or relative path="config.ini") -> (appended path=w142:path)
        n66 = call "Write NS (HMI).vi"("error in (no error)"=w148, "Message Data"=w146, "Message"="Save Para") -> ("error out"=w147:errorcluster)  [unwired: 8 in]
        n67 = call "Write Config v1.1.vi"("All Para"=w146, "file path"=w142) -> ()  [unwired: 8 in, 2 out]
      }
      frame "Manual" {
        # "Parameters"
        n68 = control-ref of="Enable Index?"() -> (w166:refnum<vi>)
        n69 = control-ref of="Enable PF?"() -> (w165:refnum<vi>)
        n70 = control-ref of="Enable Cutting?"() -> (w164:refnum<vi>)
        n71 = control-ref of="Enable Insertion?"() -> (w163:refnum<vi>)
        n72 = control-ref of="Enable TF?"() -> (w162:refnum<vi>)
        n73 = control-ref of="Enable Measure?"() -> (w160:refnum<vi>)
        n74 = Unbundle By Name(w157) -> ("Auto Para"=w156:T2)
        n75 = control-ref of="Enable Reject?"() -> (w159:refnum<vi>)
        n76 = Build Array(w166, w165, w164, w163, w162, w160, w159) -> (w161:refnum<vi>[])
        n77 = property on="Auto Para" class="Clust (strict)"("Value"=w156) -> ()  [unwired: 2 in, 2 out]
        n78 = for {
          tunnel: w161 -> [w172] mode=indexing
          n79 = property class="Bool (strict)"(reference=w172, "Val(Sgnl)"=FALSE ("Value (Signaling)")) -> ()  [unwired: 1 in, 2 out]
        }
        n80 = Unbundle By Name(w169) -> ("Main Tab"=w168:refnum<vi>)
        n81 = property class="TabCtl"(reference=w168, "Value"=Main_Tabs_v0.1."Manual Mode" ("Main Tab")) -> ()  [unwired: 1 in, 2 out]
      }
      frame "Autocycle" {
        # "Parameters"
        n82 = call "Select Model v0.1.vi"() -> ("Cancel out"=w178:bool, "Refresh Indicators?"=w175:bool, "Model out"=w179:string)  [unwired: 9 in]
        n83 = case shown="False" w178 {
          tunnel: w181 -> [w193 w208]
          tunnel: [w200 w208] -> w180
          tunnel: w179 -> [w199 _]
          tunnel: w177 -> [w196 _]
          tunnel: w176 -> [w190 _]
          tunnel: w175 -> [w183 _]
          tunnel: [w187 w207] -> w174
          tunnel: w173 -> [w184 w207]
          frame False {
            n84 = Unbundle By Name(w196) -> ("Main Tab"=w198:refnum<vi>)
            n85 = Unbundle By Name(w190) -> ("General Para 2.OutputPause"=w189:dbl, "General Para 2.RejectPause"=w188:dbl)
            n86 = call "Write NS (HMI).vi"("error in (no error)"=w193, "Message Data"=w190, "Message"="Save Para") -> ("error out"=w192:errorcluster)  [unwired: 8 in]
            n87 = property class="TabCtl"(reference=w198, "Value"=Main_Tabs_v0.1."Autocycle" ("Main Tab")) -> ()  [unwired: 1 in, 2 out]
            n88 = call "Write NS (HMI).vi"("error in (no error)"=w192, "Message Data"=w199, "Message"="Autocycle") -> ("error out"=w200:errorcluster)  [unwired: 8 in]
            n89 = property on="Home IOs" class="Bool"("Visible"=FALSE) -> ()  [unwired: 2 in, 2 out]
            n90 = property on="Back IO" class="Bool"("Visible"=TRUE) -> ()  [unwired: 2 in, 2 out]
            n91 = To Unsigned Long Integer(number=w189) -> (unsigned 32bit integer=w186:u32)
            n92 = To Unsigned Long Integer(number=w188) -> (unsigned 32bit integer=w185:u32)
            n93 = case shown="True" w183 {
              tunnel: [w202 w206] -> w187
              tunnel: w186 -> [_ w204]
              tunnel: w185 -> [_ w203]
              tunnel: w184 -> [w202 w205]
              frame False {
              }
              frame True {
                n94 = local write "GoodPause"(w204) -> ()
                n95 = local write "RejectPause"(w203) -> ()
                n96 = Bundle(cluster=w205, "GoodPause"=w204, "RejectPause"=w203) -> (w206:cluster{"GoodPause":u32, "RejectPause":u32})
              }
            }
          }
          frame True {
          }
        }
      }
      frame "Autocycle Back" {
        # "Parameters"
        n97 = Unbundle By Name(w215) -> ("Main Tab"=w214:refnum<vi>)
        n98 = property class="TabCtl"(reference=w214, "Value"=Main_Tabs_v0.1."Autocycle" ("Main Tab")) -> ()  [unwired: 1 in, 2 out]
      }
      frame "Autocycle Stats" {
        # "Parameters"
        n99 = Unbundle By Name(w222) -> ("Main Tab"=w221:refnum<vi>)
        n100 = property class="TabCtl"(reference=w221, "Value"=Main_Tabs_v0.1."Autocycle Statistics" ("Main Tab")) -> ()  [unwired: 1 in, 2 out]
      }
      frame "Autocycle IO" {
        # "Parameters"
        n101 = Unbundle By Name(w232) -> ("Main Tab"=w231:refnum<vi>)
        n102 = property class="TabCtl"(reference=w231, "Value"=Main_Tabs_v0.1."Autocycle IOs" ("Main Tab")) -> ()  [unwired: 1 in, 2 out]
        n103 = call-poly "Enqueue Message.vi"("error in (no error)"=w227, "Message"="Update IO", "Message Queue"=w225) -> ("error out"=w226:errorcluster)  [unwired: 7 in, 1 out]
      }
      frame "Update IO" {
        n104 = Unbundle By Name(w240) -> ("Main Tab"=w241:refnum<vi>)
        n105 = Wait (ms)(milliseconds to wait=u32 200) -> ()  [unwired: 1 out]
        n106 = property class="TabCtl"(reference=w241) -> ("Value"=w239:variant)  [unwired: 1 in, 2 out]
        n107 = Variant To Data(type=Main_Tabs_v0.1."Autocycle IOs" ("Main Tab"), Variant=w239) -> (data=w236:T4)  [unwired: 1 in, 1 out]
        n108 = global read "Maintenance GV.vi" "All IO"() -> (w245:T32)
        n109 = case shown="\"Autocycle IOs\"" w236 {
          tunnel: w243 -> [w253 w256]
          tunnel: [w253 w255] -> w242
          tunnel: w235 -> [_ w254]
          frame Default {
          }
          frame "Autocycle IOs" {
            n110 = call-poly "Enqueue Message.vi"("error in (no error)"=w256, "Message"="Update IO", "Message Queue"=w254) -> ("error out"=w255:errorcluster)  [unwired: 7 in, 1 out]
          }
        }
        n111 = Unbundle(w245) -> ("DI 1"=→"DI 1":T33, "DI 2"=→"DI 2":T34, "IAS 1"=→"IAS 1":dbl, "IAS 2"=→"IAS 2":dbl, "IAS 3"=→"IAS 3":dbl, "IAS 4"=→"IAS 4":dbl, "DO 1"=→"DO 1":T35)
      }
      frame "Update UI" {
        # "Update Display - Convert the message data to a string to display in the Data Display indicator."
        n112 = Variant To Data(error in=w273, type=T22 {"Array"=[], "Machine Status"=""} ("Status Cluster"), Variant=w272) -> (data=w268:T22, error out=w271:errorcluster)
        n113 = Unbundle(w268) -> ("Array"=→"Statuses":string[][], "Machine Status"=w266:string)
        "Status" <- w266
        n114 = Search and Replace String(input string=w266, search string="Autocycle is Running") -> (number of replacements=w264:i32)  [unwired: 6 in, 3 out]
        n115 = Greater Than 0?(x=w264) -> (x > 0?=w262:bool)
        n116 = Select(t=T21."Disabled and Grayed Out" ("Disabled"), s=w262, f=T21."Enabled" ("Disabled")) -> (s? t:f=w261:T21)
        n117 = property on="Home AC" class="Bool"("DisabledEnum"=w261) -> ()  [unwired: 2 in, 2 out]
        n118 = Merge Errors(w271) -> (w274:errorcluster)
      }
      frame "Autocycle Log" {
        # "Update Display - Convert the message data to a string to display in the Data Display indicator."
        n119 = Variant To Data(error in=w323, type=T24 {"Time-Stamp"=timestamp(0 s since 1904-01-01), "Auto Times"={"Index Time"=0, "TF Time"=0, "Insertion Time"=0, "Cutting Time"=0, "PF Time"=0, "Meas. Time"=0, "Reject Time"=0}, "Measurements"={"1"=0.0, "2"=0.0, "3"=0.0, "4"=0.0}, "Outputs"={"Good Parts"=0, "Reject Parts"=0}, "Cycle Time"=0.0, "Remarks"=""} ("Auto Stats"), Variant=w322) -> (data=w279:T24, error out=w321:errorcluster)
        n120 = Unbundle By Name(w279) -> ("Time-Stamp"=w317:timestamp, "Measurements"=w309:cluster{"1":dbl, "2":dbl, "3":dbl, "4":dbl}, "Outputs"=→"Output Chart":cluster{"Good Parts":u32, "Reject Parts":u32}, "Auto Times"=→"Auto Times":T9)
        "Latest Measure." <- w309
        n121 = call "Stats Unbundle.vi"("State"=Logging_FGV."Log Index", "Auto Stats"=w279) -> ("Cycle Time"=→"Cycle Time" →"Total Time":dbl, "Counters"=w313:cluster{"GoodCount":u32, "RejectCount":u32}, "OEE Cluster"=→"OEE Chart" →"OEE 2":T13, "Avg. Cycle Time"=w291:dbl, "Total Times"=w299:T36, "path"=→"path":path)  [unwired: 3 in, 1 out]
        "Avg. Time" <- w291
        n122 = Format Date/Time String(time format string (%c)="%d-%m-%Y | %H:%M:%S%3u", seconds (now)=w317) -> (date/time string=→"Timestamp":string)  [unwired: 1 in]
        n123 = Unbundle By Name(w289) -> ("Auto Para.Measur. Delays"=w288:dbl[])
        n124 = Unbundle By Name(w313) -> ("GoodCount"=w301:u32, "RejectCount"=w302:u32)
        "Rejects" <- w302
        "Good" <- w301
        "Good Count" <- w301
        "Reject Count" <- w302
        n125 = call "Auto-Pause Check.vi"("Auto Stats"=w279, "Queue"=w280, "Autopause"=w281) -> ("Autopause out"=w278:cluster{"GoodPause":u32, "RejectPause":u32})  [unwired: 8 in]
        n126 = Index Array(array=w288, index #1=1 ("index"), index #2=2 ("index")) -> (element #1=w283:dbl, element #2=w282:dbl)
        n127 = Unbundle(w299) -> ("Index"=w298:dbl, "TF"=w297:dbl, "Insert"=w296:dbl, "Cutting"=w295:dbl, "PF"=w294:dbl, "Measure."=w293:dbl, "Reject"=w292:dbl)
        n128 = Bundle("Index"=w298, "TF"=w297, "Insert"=w296, "Cutting"=w295, "PF"=w294, "Measure."=w293, "Reject"=w292, "Avg. Cycle Time"=w291) -> (→"Time Chart":T12)  [unwired: 1 in]
        n129 = Add(x=w283, y=w282) -> (x+y=w285:dbl)
        n130 = Subtract(x=w283, y=w282) -> (x-y=w284:dbl)
        n131 = Add(x=w301, y=w302) -> (x+y=→"Total Count 2":u32)
        n132 = Unbundle(w309) -> ("1"=w308:dbl, "2"=w307:dbl, "3"=w306:dbl, "4"=w305:dbl)
        n133 = Unbundle(w278) -> ("GoodPause"=→"GoodPause":u32, "RejectPause"=→"RejectPause":u32)
        n134 = Bundle("1"=w308, "2"=w307, "3"=w306, "4"=w305, w285, w284) -> (→"Measurement Chart":T37)  [unwired: 1 in]
        n135 = Merge Errors(w321) -> (w324:errorcluster)
      }
      frame "Run Manual" {
        # "Update Manual mode"
        n136 = Bundle("Manual Para"="Manual Para", "Reject Pallets"="Reject Pallets") -> (w329:T38)  [unwired: 1 in]
        n137 = for {
          tunnel: w332 -> [w340] mode=indexing
          tunnel: T21."Disabled and Grayed Out" ("Disabled") -> [w339]
          n138 = property class="Bool"(reference=w340, "DisabledEnum"=w339) -> ()  [unwired: 1 in, 2 out]
        }
        n139 = call "Write NS (HMI).vi"("error in (no error)"=w335, "Message Data"=w329, "Message"="Manual Run") -> ("error out"=w334:errorcluster)  [unwired: 8 in]
        n140 = Merge Errors(w334) -> (w337:errorcluster)
      }
      frame "Manual Status" {
        n141 = Variant To Data(error in=w369, type=T25 {"Auto Times"={"Index Time"=0, "TF Time"=0, "Insertion Time"=0, "Cutting Time"=0, "PF Time"=0, "Meas. Time"=0, "Reject Time"=0}, "Results"={"Measurements"={"1"=0.0, "2"=0.0, "3"=0.0, "4"=0.0}, "Reject Pallets"={"Reject 1"=FALSE, "Reject 2"=FALSE, "Reject 3"=FALSE, "Reject 4"=FALSE}}, "OutputCount"=0, "error out"={"status"=FALSE, "code"=0, "source"=""}} ("cluster"), Variant=w368) -> (data=w365:T25, error out=w360:errorcluster)
        n142 = Unbundle(w365) -> ("Auto Times"=w364:T9, "Results"=w356:T39, "OutputCount"=w355:u32, "error out"=w358:errorcluster)
        n143 = for {
          tunnel: w366 -> [w375] mode=indexing
          tunnel: T21."Enabled" ("Disabled") -> [w374]
          n144 = property class="Bool"(reference=w375, "DisabledEnum"=w374) -> ()  [unwired: 1 in, 2 out]
        }
        n145 = Unbundle(w356) -> ("Measurements"=w344:cluster{"1":dbl, "2":dbl, "3":dbl, "4":dbl}, "Reject Pallets"=w345:T3)
        "Measurements" <- w344
        n146 = Bundle("Auto Times"=w364, "error out"=w358) -> (→"Status 2":T10)  [unwired: 1 in]
        n147 = Bundle("Reject Pallets"=w345, "Measurements"=w344) -> (w343:T40)  [unwired: 1 in]
        n148 = call "Counts Update (manual).vi"("output cluster"=w343, "Desired Cycle Time (s)"="Ideal Time", "AVL"="AVL", "OutputCount"=w355, "Counts in"=w359) -> ("OEE"=w349:T13, "Counts out"=w354:cluster{"OutputCount":u32, "RejectCount":u32})  [unwired: 5 in]
        n149 = Unbundle(w349) -> ("PRF"=→"PRF":dbl, "QUA"=→"QUA":dbl, "OEE"=→"OEE":dbl)  [unwired: 1 out]
        n150 = Unbundle(w354) -> ("OutputCount"=→"Output Count":u32, "RejectCount"=→"Rejects 2":u32)
        n151 = case shown="True" "Continuous?" {
          tunnel: w361 -> [_ w373]
          tunnel: w358 -> [_ w372]
          frame False {
          }
          frame True {
            # "Run if continuous is TRUE & No Error"
            n152 = call-poly "Enqueue Message.vi"("error in (no error)"=w372, "Message"="Run Manual", "Message Queue"=w373) -> ()  [unwired: 7 in, 2 out]
          }
        }
      }
      frame "Reset Manual Count" {
        w378 = u32 0 ("Rejects")
        n153 = local write "Rejects 2"(w378) -> ()
        n154 = local write "Output Count"(w378) -> ()
      }
      frame "Reset AutoPause" {
        n155 = Variant To Data(error in=w391, type="" ("Message"), Variant=w389) -> (data=w387:string, error out=w390:errorcluster)
        n156 = case shown="\"ResetGoodCount\"" w387 {
          tunnel: w386 -> [w398 w403]
          tunnel: [w397 w402] -> w384
          tunnel: w385 -> [w396 w401]
          frame "ResetGoodCount" {
            n157 = Unbundle By Name(w396) -> ("General Para 2.OutputPause"=w395:dbl)
            n158 = To Unsigned Long Integer(number=w395) -> (unsigned 32bit integer=w394:u32)
            n159 = Bundle By Name(cluster=w398, "GoodPause"=w394) -> (w397:cluster{"GoodPause":u32, "RejectPause":u32})
          }
          frame "ResetRejectCount", Default {
            n160 = Unbundle By Name(w401) -> ("General Para 2.RejectPause"=w400:dbl)
            n161 = To Unsigned Long Integer(number=w400) -> (unsigned 32bit integer=w399:u32)
            n162 = Bundle By Name(cluster=w403, "RejectPause"=w399) -> (w402:cluster{"GoodPause":u32, "RejectPause":u32})
          }
        }
        n163 = Unbundle(w384) -> ("GoodPause"=w383:u32, "RejectPause"=w382:u32)
        n164 = local write "GoodPause"(w383) -> ()
        n165 = local write "RejectPause"(w382) -> ()
      }
      frame "Error" {
        w409 = 128  # call and forget
        # "Run async so that this loop will continue to run"
        # "Error"
        n166 = Variant To Data(error in=w428, type=errorcluster {"status"=FALSE, "code"=0, "source"=""} ("error constant"), Variant=w426) -> (data=w421:errorcluster, error out=w424:errorcluster)
        n167 = Unbundle By Name(w421) -> ("source"=w420:string)
        n168 = vi-ref "NewDialog.vi"() -> (w416:refnum<vi>)
        n169 = property class="VI"(reference=w416) -> (error out=w418:errorcluster, "Name"=w417:string)  [unwired: 1 in, 1 out]
        n170 = Search and Replace String(input string=w420, search string="<err>") -> (result string=w408:string)  [unwired: 6 in, 3 out]
        n171 = Open VI Reference(type specifier VI Refnum (for type only)=refnum<vi> refnum, vi path=w417, options=w409, error in (no error)=w418) -> (vi reference=w411:refnum<vi>, error out=w412:errorcluster)  [unwired: 2 in]
        n172 = call-by-ref "Start Asynchronous Call"(reference=w411, error in=w412, "inIcon"=T26."Error", "inTitle"="ERROR", "inMessage"=w408) -> (reference out=w414:refnum<vi>, error out=w413:errorcluster)  [unwired: 6 in, 3 out]
        n173 = Close Reference(reference=w414, error in (no error)=w413) -> (error out=w415:errorcluster)
        n174 = call <vilib>:"Simple Error Handler.vi"("error in (no error)"=w415) -> ()  [unwired: 4 in, 5 out]
        n175 = Merge Errors(w424) -> (w423:errorcluster)
      }
      frame "Confirm Quit" {
        # "Confirm Quit - Message that can confirm whether or not the user wants to exit the application."
        n176 = call "NewDialog.vi"("inIcon"=T26."Information", "inTitle"="SHUTDOWN?", "inButton2Text"="Shutdown", "inButton1Text"="", "inMessage"="Are you sure you want to shutdown?") -> ("outButton2"=w431:bool)  [unwired: 4 in, 2 out]
        "Shutdown?" <- w431
        n177 = case shown="True" w431 {
          tunnel: w442 -> [w443 w448]
          tunnel: [w443 w447] -> w439
          tunnel: w438 -> [_ w446]
          frame False {
          }
          frame True {
            n178 = call-poly "Enqueue Message.vi"("Priority Message? (F)"=TRUE, "error in (no error)"=w448, "Message"="Exit", "Message Queue"=w446) -> ("error out"=w447:errorcluster)  [unwired: 6 in, 1 out]
          }
        }
        n179 = Merge Errors(w439) -> (w440:errorcluster)
      }
      frame "Exit" {
        # "Stop the VI"
        # "Release the message queue reference"
        # "Exit - Exit the application."
        n180 = Variant To Data(type=errorcluster {"status"=FALSE, "code"=0, "source"=""} ("error constant"), Variant=w455) -> (data=w456:errorcluster)  [unwired: 1 in, 1 out]
        n181 = call <vilib>:"Simple Error Handler.vi"("error in (no error)"=w456) -> ()  [unwired: 4 in, 5 out]
        n182 = Send Notification(notification=TRUE, notifier=w454) -> (error out=w452:errorcluster)  [unwired: 1 in, 1 out]
        n183 = call "Fire User Event - Stop.vi"("User Event - Stop"=w460) -> ("error out"=w459:errorcluster)  [unwired: 10 in]
        n184 = Release Queue(queue=w465, error in (no error)=w458) -> (error out=w462:errorcluster)  [unwired: 1 in, 2 out]
        n185 = Merge Errors(w452, w459, w462) -> (w461:errorcluster)
      }
      frame Default {
        # "'Default' case only runs if there is a message that isn't defined in any of the other cases.  Output a programming error."
        n186 = xnode "Error Ring"("parameter 0"=w469) -> ("error out"=w470:errorcluster)
      }
    }
    n187 = call "Error Handler - Message Handling Loop.vi"("error in (no error)"=w64, "Message Queue"=w66) -> ("dup error in"=w65:errorcluster)  [unwired: 8 in, 1 out]
  }
  n188 = while {
    tunnel: w34 -> [w487]
    shift-right: [w485] -> w40
    shift-left: w37 -> [w486]
    tunnel: [w481] -> w38
    tunnel: w3 -> [w479]
    stop <- w483 stop-if-true
    # "Event Handling Loop"
    n189 = event shown="[13] \"ResetGoodCount\", \"ResetRejectCount\": Value Change" {
      selector: w486 -> [_ _ _ _ _ _ _ _ _ _ _ _ _ _ _ _ _ _ _ _ _]
      dyn-events: [_ _ _ _ _ _ _ _ _ _ _ _ _ _ _ _ _ _ _ _ _] -> w485
      timeout: 500 -> [_ _ _ _ _ _ _ _ _ _ _ _ _ _ _ _ _ _ _ _ _]
      tunnel: [_ _ _ _ _ _ _ _ _ _ _ _ _ _ _ _ _ _ _ _ TRUE ("Discard?")] -> w483
      tunnel: w487 -> [w492 w496 w508 w513 w517 w521 w525 w529 w534 w539 w548 w572 w576 w580 w585 w587 w590 w621 w630 w639 w641]
      tunnel: [w491 _ _ w512 w516 w520 w524 w528 w533 w538 w547 w573 _ _ w583 w588 w593 _ _ _ _] -> w484
      tunnel: [w490 w496 w508 w511 w515 w519 w523 w527 w532 w537 w546 w572 w576 w580 w584 w587 w589 w621 w630 w639 w641] -> w482
      tunnel: w479 -> [_ _ _ _ _ _ _ _ _ _ w540 _ _ _ _ _ _ _ _ _ _]
      event Panel Close? {
        n190 = event-data() -> ()  [unwired: 1 in, 1 out]
        n191 = call-poly "Enqueue Message.vi"("Priority Message? (F)"=TRUE, "Message"="Exit", "Message Queue"=w492) -> ("error out"=w491:errorcluster, "dup Message Queue"=w490:refnum<queue>)  [unwired: 7 in]
        n192 = event-data("Discard?"=TRUE) -> ()  [unwired: 1 in, 1 out]
      }
      event Timeout {
        n193 = event-data() -> ()  [unwired: 1 in, 1 out]
        n194 = Format Date/Time String(time format string (%c)="%d %b %Y | %I:%M:%S %p") -> (date/time string=→"Date-Time":string)  [unwired: 2 in]
      }
      event "View Log": Value Change {
        w507 = 128  # call and forget
        n195 = event-data() -> ()  [unwired: 1 in, 1 out]
        n196 = local read "path"() -> (w497:path)
        n197 = vi-ref "View Log.vi"() -> (w500:refnum<vi>)
        n198 = property class="VI"(reference=w500) -> (error out=w498:errorcluster, "Name"=w499:string)  [unwired: 1 in, 1 out]
        n199 = Open VI Reference(type specifier VI Refnum (for type only)=refnum<vi> refnum, vi path=w499, options=w507, error in (no error)=w498) -> (vi reference=w505:refnum<vi>, error out=w504:errorcluster)  [unwired: 2 in]
        n200 = call-by-ref "Start Asynchronous Call"(reference=w505, error in=w504, "file path"=w497) -> (reference out=w502:refnum<vi>, error out=w503:errorcluster)  [unwired: 10 in, 1 out]
        n201 = Close Reference(reference=w502, error in (no error)=w503) -> (error out=w501:errorcluster)
        n202 = call <vilib>:"Simple Error Handler.vi"("error in (no error)"=w501) -> ()  [unwired: 4 in, 5 out]
      }
      event "Shutdown": Value Change {
        n203 = event-data() -> ()  [unwired: 1 in, 1 out]
        n204 = call-poly "Enqueue Message.vi"("Priority Message? (F)"=TRUE, "Message"="Confirm Quit", "Message Queue"=w513) -> ("error out"=w512:errorcluster, "dup Message Queue"=w511:refnum<queue>)  [unwired: 7 in]
      }
      event "Home Para", "Home Manual", "Home IOs": Value Change {
        n205 = event-data() -> ()  [unwired: 1 in, 1 out]
        n206 = call-poly "Enqueue Message.vi"("Message"="Initialize", "Message Queue"=w517) -> ("error out"=w516:errorcluster, "dup Message Queue"=w515:refnum<queue>)  [unwired: 8 in]
      }
      event "Back Stats", "Back IO": Value Change {
        n207 = event-data() -> ()  [unwired: 1 in, 1 out]
        n208 = call-poly "Enqueue Message.vi"("Message"="Autocycle Back", "Message Queue"=w521) -> ("error out"=w520:errorcluster, "dup Message Queue"=w519:refnum<queue>)  [unwired: 8 in]
      }
      event "Stats": Value Change {
        n209 = event-data() -> ()  [unwired: 1 in, 1 out]
        n210 = call-poly "Enqueue Message.vi"("Message"="Autocycle Stats", "Message Queue"=w525) -> ("error out"=w524:errorcluster, "dup Message Queue"=w523:refnum<queue>)  [unwired: 8 in]
      }
      event "All IO", "All IOs": Value Change {
        n211 = event-data() -> ()  [unwired: 1 in, 1 out]
        n212 = call-poly "Enqueue Message.vi"("Message"="Autocycle IO", "Message Queue"=w529) -> ("error out"=w528:errorcluster, "dup Message Queue"=w527:refnum<queue>)  [unwired: 8 in]
      }
      event "Home AC": Value Change {
        n213 = event-data() -> ()  [unwired: 1 in, 1 out]
        n214 = call-poly "Enqueue Message.vi"("Message"="Initialize", "Message Queue"=w534) -> ("error out"=w533:errorcluster, "dup Message Queue"=w532:refnum<queue>)  [unwired: 8 in]
        n215 = call "Write NS (HMI).vi"("Message"="Exit Autocycle") -> ()  [unwired: 10 in, 1 out]
      }
      event "Maintenance", "Manual": Value Change {
        n216 = event-data() -> ("CtlRef"=w536:refnum<vi>)  [unwired: 1 in]
        n217 = property class="Bool"(reference=w536) -> ("Label.Text"=w535:string)  [unwired: 1 in, 2 out]
        n218 = call-poly "Enqueue Message.vi"("Message"=w535, "Message Queue"=w539) -> ("error out"=w538:errorcluster, "dup Message Queue"=w537:refnum<queue>)  [unwired: 8 in]
      }
      event "Parameters": Value Change {
        n219 = event-data() -> ("CtlRef"=w545:refnum<vi>)  [unwired: 1 in, 2 out]
        n220 = call "HMI Pop Up Num KP v1.1.vi"("Password Display (F)"=FALSE, "Message In"="Please enter the passcode below:") -> ("Canceled"=w542:bool, "String Out"=w541:string)  [unwired: 8 in]
        n221 = case shown="False" w542 {
          tunnel: w548 -> [w555 w567]
          tunnel: [w554 _] -> w547
          tunnel: [w553 w567] -> w546
          tunnel: w545 -> [w552 _]
          tunnel: w541 -> [w551 _]
          tunnel: w540 -> [w550 _]
          frame False {
            n222 = Equal?(x=w551, y=w550) -> (x = y?=w549:bool)
            n223 = case shown="False" w549 {
              tunnel: w555 -> [w560 w565]
              tunnel: [w559 w564] -> w554
              tunnel: [w558 w563] -> w553
              tunnel: w552 -> [w557 _]
              frame True {
                n224 = property class="Bool"(reference=w557) -> ("Label.Text"=w556:string)  [unwired: 1 in, 2 out]
                n225 = call-poly "Enqueue Message.vi"("Message"=w556, "Message Queue"=w560) -> ("error out"=w559:errorcluster, "dup Message Queue"=w558:refnum<queue>)  [unwired: 8 in]
              }
              frame False {
                n226 = xnode "Error Ring"() -> ("error out"=w561:errorcluster)
                n227 = call-poly "Enqueue Message.vi"("Message Data"=w561, "Message"="Error" ("Message In"), "Message Queue"=w565) -> ("error out"=w564:errorcluster, "dup Message Queue"=w563:refnum<queue>)  [unwired: 7 in]
              }
            }
          }
          frame True {
          }
        }
      }
      event "End Cycle", "Enable Cutting?", "Enable TF?", "Enable PF?", "Enable Index?", "Enable Measure?", "Enable Reject?", "Enable Agitate?", "Enable BF?", "Enable Insertion?": Value Change {
        n228 = event-data() -> ("CtlRef"=w574:refnum<vi>, "NewVal"=w568:bool)  [unwired: 1 in, 1 out]
        n229 = property class="Bool"(reference=w574) -> ("Label.Text"=w571:string)  [unwired: 1 in, 2 out]
        n230 = Concatenate Strings("GV:" ("string"), w571) -> (w569:string)
        n231 = call "Write NS (HMI).vi"("Message Data"=w568, "Message"=w569) -> ("error out"=w573:errorcluster)  [unwired: 9 in]
      }
      event "Reset MCount": Value Change {
        n232 = event-data() -> ()  [unwired: 1 in, 6 out]
        n233 = call-poly "Enqueue Message.vi"("Message"="Reset Manual Count", "Message Queue"=w576) -> ()  [unwired: 8 in, 2 out]
      }
      event "ResetGoodCount", "ResetRejectCount": Value Change {
        n234 = event-data() -> ("CtlRef"=w578:refnum<vi>)  [unwired: 1 in]
        n235 = property class="Bool"(reference=w578) -> ("Label.Text"=w577:string)  [unwired: 1 in, 2 out]
        n236 = call-poly "Enqueue Message.vi"("Message Data"=w577, "Message"="Reset AutoPause", "Message Queue"=w580) -> ()  [unwired: 7 in, 2 out]
      }
      event "Run Manual": Value Change {
        n237 = event-data() -> ("CtlRef"=w582:refnum<vi>)  [unwired: 1 in, 2 out]
        n238 = property class="Bool"(reference=w582) -> ("Label.Text"=w581:string)  [unwired: 1 in, 2 out]
        n239 = call-poly "Enqueue Message.vi"("Message"=w581, "Message Queue"=w585) -> ("error out"=w583:errorcluster, "dup Message Queue"=w584:refnum<queue>)  [unwired: 8 in]
      }
      event "Toggle Motor": Value Change {
        n240 = event-data() -> ()  [unwired: 1 in, 3 out]
        n241 = call "Write NS (HMI).vi"("Message"="Toggle Motor") -> ("error out"=w588:errorcluster)  [unwired: 10 in]
      }
      event "Save Para": Value Change {
        n242 = event-data() -> ()  [unwired: 1 in, 3 out]
        n243 = Cluster To Array(cluster="Agitator Para") -> (array=w610:u32[])
        n244 = Cluster To Array(cluster="Tube Feeder Para") -> (array=w608:u32[])
        n245 = Cluster To Array(cluster="Insertion Para") -> (array=w606:u32[])
        n246 = Cluster To Array(cluster="Cutting Para") -> (array=w604:u32[])
        n247 = Cluster To Array(cluster="PF Para") -> (array=w602:u32[])
        n248 = Cluster To Array(cluster="Meas. Para") -> (array=w600:dbl[])
        n249 = Cluster To Array(cluster="Reject Para") -> (array=w598:u32[])
        n250 = Cluster To Array(cluster="BF Para") -> (array=w596:u32[])
        n251 = Bundle By Name(cluster=T2 {"Agitator Delays"=[1000], "TF Delays"=[1000], "Insertion Delays"=[1000], "Cutting Delays"=[1000], "PF Delays"=[1000], "Measur. Delays"=[1000.0], "Reject Delays"=[1000], "BF Delays"=[1000]} ("Auto Para"), "Agitator Delays"=w610, "TF Delays"=w608, "Insertion Delays"=w606, "Cutting Delays"=w604, "PF Delays"=w602, "Measur. Delays"=w600, "Reject Delays"=w598, "BF Delays"=w596) -> (w595:T2)
        n252 = Bundle("Auto Para"=w595, "General Para"="General Para") -> (w592:cluster{"Auto Para":T2, "General Para":T1})  [unwired: 1 in]
        n253 = property on="Auto Para" class="Clust (strict)"("Value"=w595) -> ()  [unwired: 2 in, 2 out]
        n254 = call-poly "Enqueue Message.vi"("Message Data"=w592, "Message"="Update Para", "Message Queue"=w590) -> ("error out"=w593:errorcluster, "dup Message Queue"=w589:refnum<queue>)  [unwired: 7 in]
      }
      event "Insertion Para.Delay 1", "Insertion Para.Delay 2", "Agitator Para.Delay 1", "Agitator Para.Delay 2", "Cutting Para.Delay", "Cutting Para.Delay 2", "Cutting Para.Delay 3", "Tube Feeder Para.Delay", "Tube Feeder Para.Delay 2", "Tube Feeder Para.Max Attempts", "PF Para.Delay 1", "PF Para.Delay 2", "Reject Para.Delay", "BF Para.Delay 1", "BF Para.Delay 2", "Tube Feeder Para.Timeout": Mouse Up {
        n255 = event-data() -> ("CtlRef"=w613:refnum<vi>)  [unwired: 1 in, 4 out]
        n256 = property class="DigNum (strict)"(reference=w613) -> (reference out=w616:refnum<vi>, "Value"=w617:u32)  [unwired: 1 in, 1 out]
        n257 = Number To Fractional String(number=w617, precision (6)=0.0 ("width (-)")) -> (F-format string=w615:string)  [unwired: 2 in]
        n258 = call "HMI Pop Up Num KP v1.1.vi"("String In"=w615) -> ("String Out"=w614:string)  [unwired: 9 in, 1 out]
        n259 = Fract/Exp String To Number(string=w614, default (0 dbl)=0.0 ("default (0 I32)")) -> (number=w619:dbl)  [unwired: 2 in, 1 out]
        n260 = property class="DigNum (strict)"(reference=w616, "Value"=w619) -> ()  [unwired: 1 in, 2 out]
      }
      event "Meas. Para.Delay": Mouse Up {
        n261 = event-data() -> ("CtlRef"=w622:refnum<vi>)  [unwired: 1 in, 4 out]
        n262 = property class="DigNum (strict)"(reference=w622) -> (reference out=w625:refnum<vi>, "Value"=w626:dbl)  [unwired: 1 in, 1 out]
        n263 = Number To Fractional String(number=w626, precision (6)=0.0 ("width (-)")) -> (F-format string=w624:string)  [unwired: 2 in]
        n264 = call "HMI Pop Up Num KP v1.1.vi"("String In"=w624) -> ("String Out"=w623:string)  [unwired: 9 in, 1 out]
        n265 = Fract/Exp String To Number(string=w623, default (0 dbl)=0.0 ("default (0 I32)")) -> (number=w628:dbl)  [unwired: 2 in, 1 out]
        n266 = property class="DigNum (strict)"(reference=w625, "Value"=w628) -> ()  [unwired: 1 in, 2 out]
      }
      event "Meas. Para.Mean Length", "Meas. Para.Tolerance": Mouse Up {
        n267 = event-data() -> ("CtlRef"=w631:refnum<vi>)  [unwired: 1 in, 4 out]
        n268 = property class="DigNum (strict)"(reference=w631) -> (reference out=w634:refnum<vi>, "Value"=w635:dbl)  [unwired: 1 in, 1 out]
        n269 = Number To Fractional String(number=w635, precision (6)=2.0 ("width (-)")) -> (F-format string=w633:string)  [unwired: 2 in]
        n270 = call "HMI Pop Up Num KP v1.1.vi"("String In"=w633) -> ("String Out"=w632:string)  [unwired: 9 in, 1 out]
        n271 = Fract/Exp String To Number(string=w632, default (0 dbl)=0.0 ("default (0 I32)")) -> (number=w637:dbl)  [unwired: 2 in, 1 out]
        n272 = property class="DigNum (strict)"(reference=w634, "Value"=w637) -> ()  [unwired: 1 in, 2 out]
      }
      event User Event {
        # "The Message Handling Loop processed an \"Exit\" message, which fired this event to stop the Event Handling Loop."
        n273 = event-data() -> ()  [unwired: 1 in, 1 out]
      }
    }
    n274 = call "Error Handler - Event Handling Loop.vi"("error in (no error)"=w484, "Message Queue"=w482) -> ("dup error in"=w481:errorcluster)  [unwired: 8 in, 1 out]
  }
  n275 = call "HMI-cRIO Connection Manager.vi"("error in"=w2, "notifier in"=w8, "Queue in"=w34) -> ("error out"=w28:errorcluster, "Notifier out"=w29:refnum<notifier>)  [unwired: 7 in]
  n276 = Unregister For Events(event registration refnum=w40, error in=w38) -> (error out=w41:errorcluster)
  n277 = Merge Errors(w41, w43, w28) -> (w42:errorcluster)
  n278 = call "Destroy User Event - Stop.vi"("error in (no error)"=w42, "User Event - Stop"=w36) -> ("error out"=w31:errorcluster)  [unwired: 9 in]
  n279 = Release Notifier(notifier=w29, error in (no error)=w31) -> (error out=w30:errorcluster)  [unwired: 1 in, 2 out]
  n280 = disable-structure shown="RUN_TIME_ENGINE==True" {
    disable-tunnel: w30 -> [_ _]
    frame condition #0 (active) {
    }
    frame condition #1 {
      n281 = local read "Shutdown?"() -> (w642:bool)
      n282 = case shown="True" w642 {
        tunnel: [_ w644] -> w643
        frame False {
        }
        frame True {
          n283 = call <vilib>:"System Exec.vi"("wait until completion? (T)"=TRUE, "command line"="Shutdown -s -f -t 10") -> ("error out"=w644:errorcluster)  [unwired: 6 in, 3 out]
        }
      }
      n284 = flat-sequence {
        tunnel: w643 -> [_]
        frame #0 {
          n285 = Quit LabVIEW() -> ()  [unwired: 1 in]
        }
      }
    }
  }
